vi "NF90 Serial Port Init.vi"(0 "port number":refnum<visa-resource-name>, 7 "data bits":u16=7 min=5 max=8 step=1, 11 "parity":u16(ring)=2 items=["no parity", "odd parity", "even parity", "mark parity", "space parity"]) -> (4 "port number":refnum<visa-resource-name>, 15 "error out":errorcluster)   [LabVIEW 2015]
doc: "Initializes the selected serial port to the specified settings."
uses:
  <vilib>/Instr/_visa.llb/VISA Configure Serial Port (Instr).vi
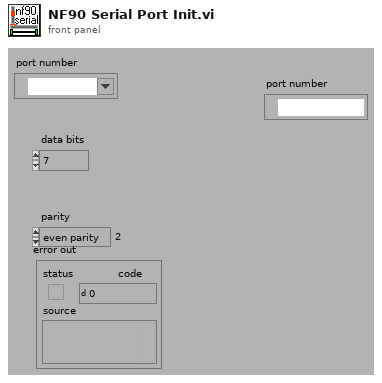
[diagram p1: front panel]
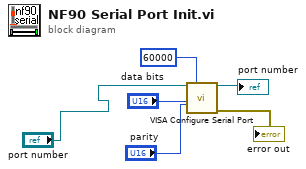
[diagram p0: block diagram]
diagram:
  n1 = call-poly "VISA Configure Serial Port"("VISA resource name"="port number", "timeout (10sec)"=u32 60000, "data bits (8)"="data bits", "parity (0:none)"="parity") -> ("VISA resource name out"=→"port number":refnum<visa-resource-name>, "error out"=→"error out":errorcluster)  [unwired: 10 in]
